vi "Initialize Parent STEP Class Values.vi"(8 "error in (no error)":errorcluster, 11 "STEP in":refnum<class "STEP.lvclass">) -> (0 "error out":errorcluster, 3 "STEP out":refnum<class "STEP.lvclass">)   [LabVIEW 2014, in "SeqLoop.lvlib" / "STEP Classes.lvlib" / "STEP.lvclass"]
uses:
  STEP.lvclass
  TypeDefs/LogicParsedExpression.ctl
  Mimico Display/TypeDefs/Mimic Data.ctl
  Mimico Display/TypeDefs/BG Image.ctl
  Mimico Display/TypeDefs/mObject.ctl
  STEP.lvclass/STEP.ctl
  SeqLoop.lvlib
  Mimico Display/Mimico Display.lvlib
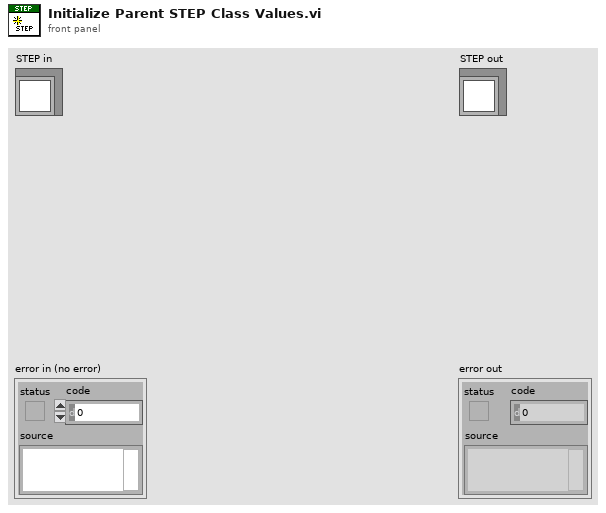
[diagram p1: front panel]
types:
  T1 = cluster{"jump?":bool, "Initial STEP":u32, "Number of STEPs":u32, "Repetitions":u32, "Reset?":bool}
  T2 = typedef "SeqLoop.lvlib/Mimico Display.lvlib/Mimic Data.ctl" = cluster{"BG Image":T3, "Mimic mObjects":T4[]}
  T3 = typedef "SeqLoop.lvlib/Mimico Display.lvlib/BG Image.ctl" = cluster{"Path":path, "point":cluster{"x":i16, "y":i16}}
  T4 = typedef "SeqLoop.lvlib/Mimico Display.lvlib/mObject.ctl" = cluster{"point":cluster{"x":i16, "y":i16}, "Precision (Digits)":i32, "Visible?":bool, "Ref":string, "Comment":string}
  T5 = typedef "SeqLoop.lvlib/LogicParsedExpression.ctl" = cluster{"RPN ":string[], "Variables":string[], "Ctes":string[], "Formula":string, "Message":string}
  T6 = cluster{"Advance":T5, "Error ":T5, "Alarm 1":T5, "Alarm 2":T5, "Alarm 3":T5, "Alarm 4":T5}
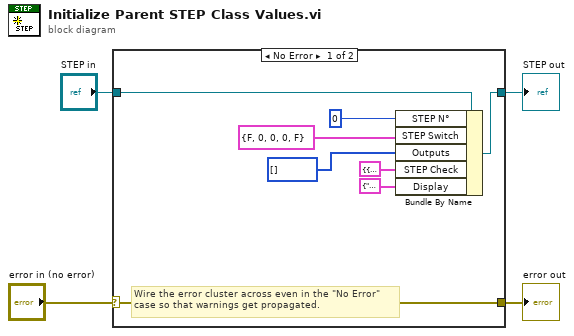
[diagram p0: block diagram]
diagram:
  n1 = case shown="No Error" "error in (no error)" {
    selector: "error in (no error)" -> [w12 w14]
    tunnel: [w12 w14] -> w3
    tunnel: [w10 w13] -> w1
    tunnel: "STEP in" -> [w11 w13]
    frame No Error {
      # "Wire the error cluster across even in the \"No Error\"\ncase so that warnings get propagated."
      n2 = Bundle By Name(cluster=w11, "STEP N°"=u32 0, "STEP Switch"=T1 {"jump?"=FALSE, "Initial STEP"=0, "Number of STEPs"=0, "Repetitions"=0, "Reset?"=FALSE}, "Outputs"=i32[] [], "STEP Check"=T6 {"Advance"={"RPN "=[], "Variables"=[], "Ctes"=[], "Formula"="", "Message"=""}, "Error "={"RPN "=[], "Variables"=[], "Ctes"=[], "Formula"="", "Message"=""}, "Alarm 1"={"RPN "=[], "Variables"=[], "Ctes"=[], "Formula"="", "Message"=""}, "Alarm 2"={"RPN "=[], "Variables"=[], "Ctes"=[], "Formula"="", "Message"=""}, "Alarm 3"={"RPN "=[], "Variables"=[], "Ctes"=[], "Formula"="", "Message"=""}, "Alarm 4"={"RPN "=[], "Variables"=[], "Ctes"=[], "Formula"="", "Message"=""}}, "Display"=cluster{"Mssg Op":string, "Mimic Data":T2} {"Mssg Op"="", "Mimic Data"={"BG Image"={"Path"=path "", "point"={"x"=0, "y"=0}}, "Mimic mObjects"=[]}}) -> (w10:refnum<class "STEP.lvclass">)
    }
    frame Error {
    }
  }
  "error out" <- w3
  "STEP out" <- w1
